vi "sub vi - calibration v1.vi"() -> ()   [LabVIEW 2013]
uses:
  <vilib>/Platform/TimedLoop/XDataNode/timing_clust.ctl
  <vilib>/Platform/TimedLoop/XDataNode/nitl_modes.ctl
  <vilib>/Platform/TimedLoop/XDataNode/wakeup.ctl
  <vilib>/platform/TimedLoop/XDataNode/XDataNode.xnode
  <vilib>/Platform/TimedLoop/XDataNode/XDNodeRunTimeDep.lvlib
panel:
  out "UPDATE":bool
  in  "stop":bool
  in  "Tab Control":T1(tab)
  out "LAB01-1 (GRAPH)":dynamicdata(graph)
  out "LAB01-2 (GRAPH)":dynamicdata(graph)
  in  "LAB01 (CAL)":T2 {"2 (TN) cal" min=0.0 step=0.01 format="%.2f"; "2 (TL) cal" min=0.0 step=0.01 format="%.2f"; "2 (PF) cal" min=0.0 step=0.01 format="%.2f"; "2 (V) cal" min=0.0 step=0.01 format="%.2f"; "2 (A) cal" min=0.0 step=0.01 format="%.2f"; "1 (TN) cal" min=0.0 step=0.01 format="%.2f"; "1 (TL) cal" min=0.0 step=0.01 format="%.2f"; "1 (PF) cal" min=0.0 step=0.01 format="%.2f"; "1 (V) cal" min=0.0 step=0.01 format="%.2f"; "1  (A) cal" min=0.0 step=0.01 format="%.2f"}
  out "LAB01 (SIGNALS)":T3 {"2 (PF)" format="%.2f"; "2 (A)" format="%.1f"; "1 (PF)" format="%.2f"; "1 (A)" format="%.1f"}
  out "LAB02 (SIGNALS)":T3 {"2 (PF)" format="%.2f"; "2 (A)" format="%.1f"; "1 (PF)" format="%.2f"; "1 (A)" format="%.1f"}
  in  "LAB02 (CAL)":T4 {"2 (TN) cal" min=0.0 step=0.01 format="%.2f"; "2 (TL) cal" min=0.0 step=0.01 format="%.2f"; "2 (PF) cal" min=0.0 step=0.01 format="%.2f"; "2 (V) cal" min=0.0 step=0.01 format="%.2f"; "2 (A) cal" min=0.0 step=0.01 format="%.2f"; "1 (TN) cal" min=0.0 step=0.01 format="%.2f"; "1 (TL) cal" min=0.0 step=0.01 format="%.2f"; "1 (PF) cal" min=0.0 step=0.01 format="%.2f"; "1 (V) cal" min=0.0 step=0.01 format="%.2f"; "1 (A) cal" min=0.0 step=0.01 format="%.2f"}
  out "LAB02-2 (GRAPH)":dynamicdata(graph)
  out "LAB02-1 (GRAPH)":dynamicdata(graph)
  out "LAB03 (SIGNALS)":T3 {"2 (PF)" format="%.2f"; "2 (A)" format="%.1f"; "1 (PF)" format="%.2f"; "1 (A)" format="%.1f"}
  in  "LAB03 (CAL)":T2 {"2 (TN) cal" min=0.0 step=0.01 format="%.2f"; "2 (TL) cal" min=0.0 step=0.01 format="%.2f"; "2 (PF) cal" min=0.0 step=0.01 format="%.2f"; "2 (V) cal" min=0.0 step=0.01 format="%.2f"; "2 (A) cal" min=0.0 step=0.01 format="%.2f"; "1 (TN) cal" min=0.0 step=0.01 format="%.2f"; "1 (TL) cal" min=0.0 step=0.01 format="%.2f"; "1 (PF) cal" min=0.0 step=0.01 format="%.2f"; "1 (V) cal" min=0.0 step=0.01 format="%.2f"; "1  (A) cal" min=0.0 step=0.01 format="%.2f"}
  out "LAB03-2 (GRAPH)":dynamicdata(graph)
  out "LAB03-1 (GRAPH)":dynamicdata(graph)
  out "LAB04 (SIGNALS)":T3 {"2 (PF)" format="%.2f"; "2 (A)" format="%.1f"; "1 (PF)" format="%.2f"; "1 (A)" format="%.1f"}
  in  "LAB04 (CAL)":T2 {"2 (TN) cal" min=0.0 step=0.01 format="%.2f"; "2 (TL) cal" min=0.0 step=0.01 format="%.2f"; "2 (PF) cal" min=0.0 step=0.01 format="%.2f"; "2 (V) cal" min=0.0 step=0.01 format="%.2f"; "2 (A) cal" min=0.0 step=0.01 format="%.2f"; "1 (TN) cal" min=0.0 step=0.01 format="%.2f"; "1 (TL) cal" min=0.0 step=0.01 format="%.2f"; "1 (PF) cal" min=0.0 step=0.01 format="%.2f"; "1 (V) cal" min=0.0 step=0.01 format="%.2f"; "1  (A) cal" min=0.0 step=0.01 format="%.2f"}
  out "LAB04-2 (GRAPH)":dynamicdata(graph)
  out "LAB04-1 (GRAPH)":dynamicdata(graph)
  out "LAB05 (SIGNALS)":T3 {"2 (PF)" format="%.2f"; "2 (A)" format="%.1f"; "1 (PF)" format="%.2f"; "1 (A)" format="%.1f"}
  in  "LAB05 (CAL)":T2 {"2 (TN) cal" min=0.0 step=0.01 format="%.2f"; "2 (TL) cal" min=0.0 step=0.01 format="%.2f"; "2 (PF) cal" min=0.0 step=0.01 format="%.2f"; "2 (V) cal" min=0.0 step=0.01 format="%.2f"; "2 (A) cal" min=0.0 step=0.01 format="%.2f"; "1 (TN) cal" min=0.0 step=0.01 format="%.2f"; "1 (TL) cal" min=0.0 step=0.01 format="%.2f"; "1 (PF) cal" min=0.0 step=0.01 format="%.2f"; "1 (V) cal" min=0.0 step=0.01 format="%.2f"; "1  (A) cal" min=0.0 step=0.01 format="%.2f"}
  out "LAB05-2 (GRAPH)":dynamicdata(graph)
  out "LAB05-1 (GRAPH)":dynamicdata(graph)
  out "Temperature data error":bool
  out "file error out":errorcluster
  out "Analog Loop Time":dbl
  out "analog read ERROR":errorcluster[](array[cluster])
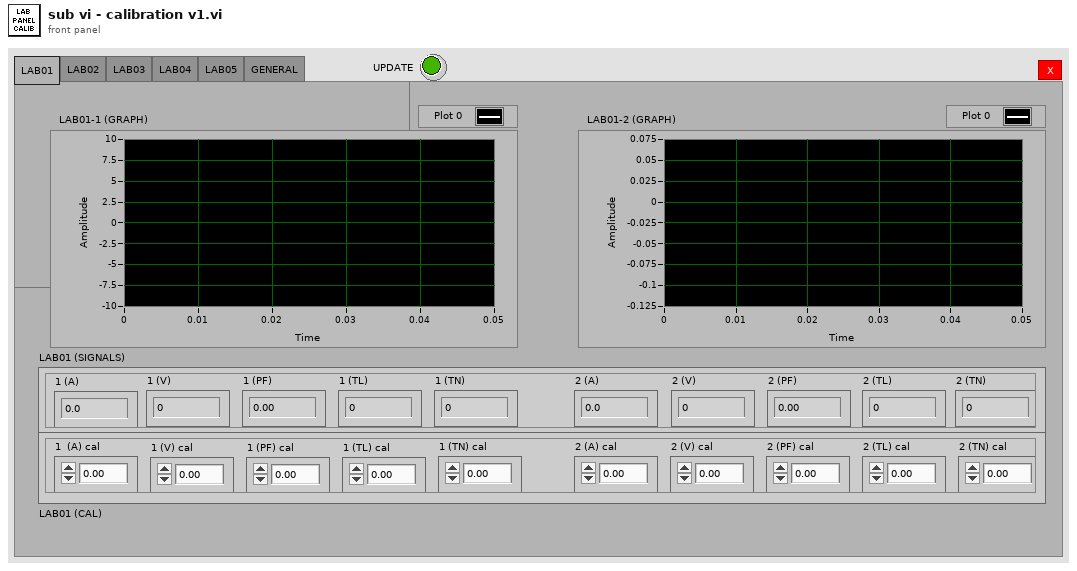
[diagram p1: front panel]
types:
  T1 = enum32{"LAB01", "LAB02", "LAB03", "LAB04", "LAB05", "GENERAL"}
  T2 = cluster{"1  (A) cal":dbl, "1 (V) cal":dbl, "1 (PF) cal":dbl, "1 (TL) cal":dbl, "1 (TN) cal":dbl, "2 (A) cal":dbl, "2 (V) cal":dbl, "2 (PF) cal":dbl, "2 (TL) cal":dbl, "2 (TN) cal":dbl}
  T3 = cluster{"1 (TL)":dbl, "1 (TN)":dbl, "2 (TL)":dbl, "2 (TN)":dbl, "1 (A)":dbl, "1 (V)":dbl, "1 (PF)":dbl, "2 (A)":dbl, "2 (V)":dbl, "2 (PF)":dbl}
  T4 = cluster{"1 (A) cal":dbl, "1 (V) cal":dbl, "1 (PF) cal":dbl, "1 (TL) cal":dbl, "1 (TN) cal":dbl, "2 (A) cal":dbl, "2 (V) cal":dbl, "2 (PF) cal":dbl, "2 (TL) cal":dbl, "2 (TN) cal":dbl}
  T5 = enum16{"open", "replace", "create", "open or create", "replace or create", "replace or create with confirmation"}
  T6 = typedef "XDNodeRunTimeDep.lvlib/timing_clust.ctl" = cluster{"Expected End [f-1]":u64, "Actual End [f-1]":u64, "Finished Late? [f-1]":bool, "Expected End [i-1]":u64, "Actual End [i-1]":u64, "Finished Late? [i-1]":bool, "Expected Start [i]":u64, "Actual Start [i]":u64, "Expected Start [f]":u64, "Actual Start [f]":u64, "Source Name":string, "Structure Name":string, "Period":i64, "Deadline":i64, "Offset":i64, "Start":i64, "Priority":i32, "Timeout":i32, "Mode":T7, "Wakeup Reason":T8, "Error":errorcluster, "Source Type":string, "Secondary Source Type":string, "Global End Time":u64, "Global Start Time":u64, "Frame Duration":u64, "Iteration Duration":u64, "Assigned CPU":i32, "I/O Scan Engine Mode":u32}
  T7 = typedef "XDNodeRunTimeDep.lvlib/nitl_modes.ctl" = enum32{"No Change", "Process missed periods, maintain original phase", "Discard missed periods, maintain original phase", "Process missed periods, ignore original phase", "Discard missed periods, ignore original phase"}
  T8 = typedef "XDNodeRunTimeDep.lvlib/wakeup.ctl" = enum32{"Normal", "Aborted", "Asynchronous wakeup", "Timing source error", "Timed loop error", "Timeout"}
  T9 = cluster{"LAB01-1 (A)":dbl, "LAB01-1 (V)":dbl, "LAB01-1 (PF)":dbl, "LAB01-2 (A)":dbl, "LAB01-2 (V)":dbl, "LAB01-2 (PF)":dbl}
  T10 = cluster{"LAB02-1 (A)":dbl, "LAB02-1 (V)":dbl, "LAB02-1 (PF)":dbl, "LAB02-2 (A)":dbl, "LAB02-2 (V)":dbl, "LAB02-2 (PF)":dbl}
  T11 = cluster{"LAB03-1 (A)":dbl, "LAB03-1 (V)":dbl, "LAB03-1 (PF)":dbl, "LAB03-2 (A)":dbl, "LAB03-2 (V)":dbl, "LAB03-2 (PF)":dbl}
  T12 = cluster{"LAB04-1 (A)":dbl, "LAB04-1 (V)":dbl, "LAB04-1 (PF)":dbl, "LAB04-2 (A)":dbl, "LAB04-2 (V)":dbl, "LAB04-2 (PF)":dbl}
  T13 = cluster{"LAB05-1 (A)":dbl, "LAB05-1 (V)":dbl, "LAB05-1 (PF)":dbl, "LAB05-2 (A)":dbl, "LAB05-2 (V)":dbl, "LAB05-2 (PF)":dbl}
  T14 = cluster{"T1":dbl, "T2":dbl, "T3":dbl, "T4":dbl, "ID":dbl, "ER":dbl}
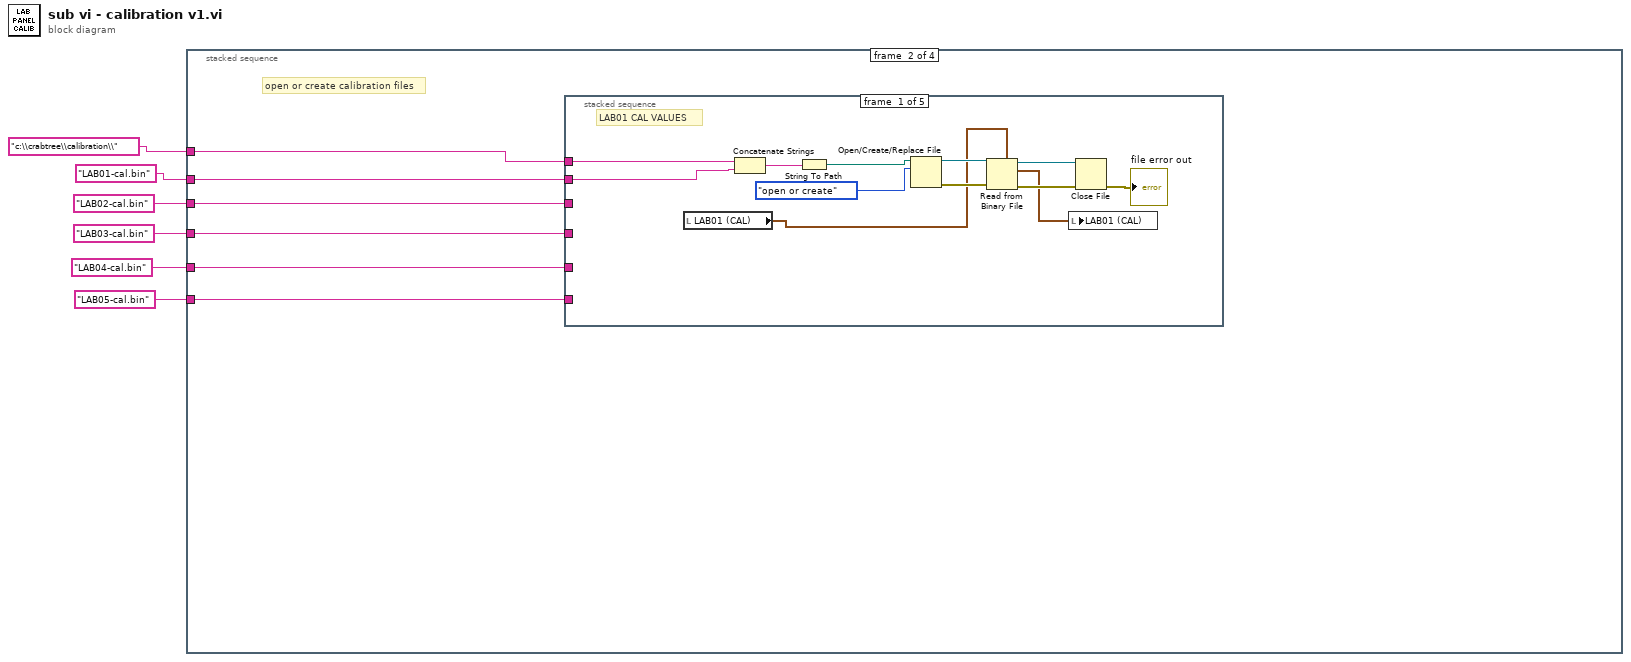
[diagram p0: block diagram]
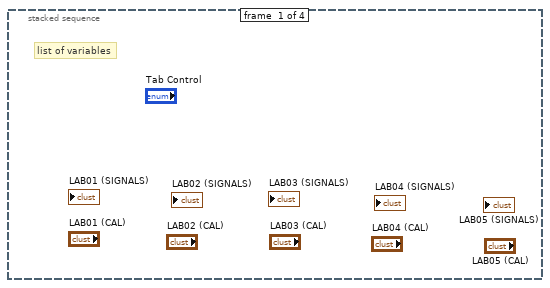
[diagram p2: hidden frame]
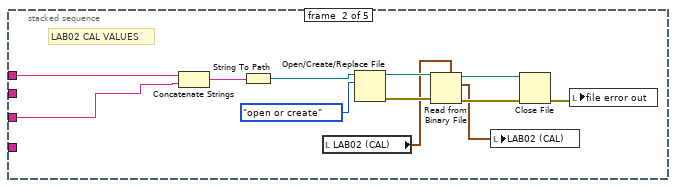
[diagram p3: hidden frame]
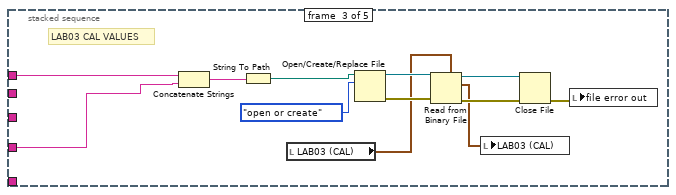
[diagram p4: hidden frame]
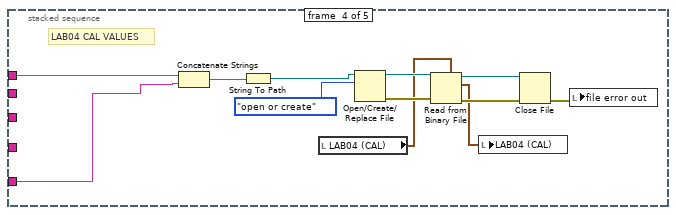
[diagram p5: hidden frame]
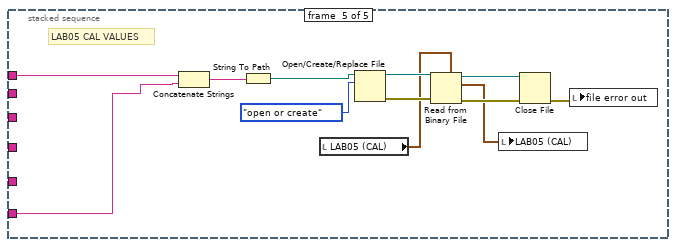
[diagram p6: hidden frame]
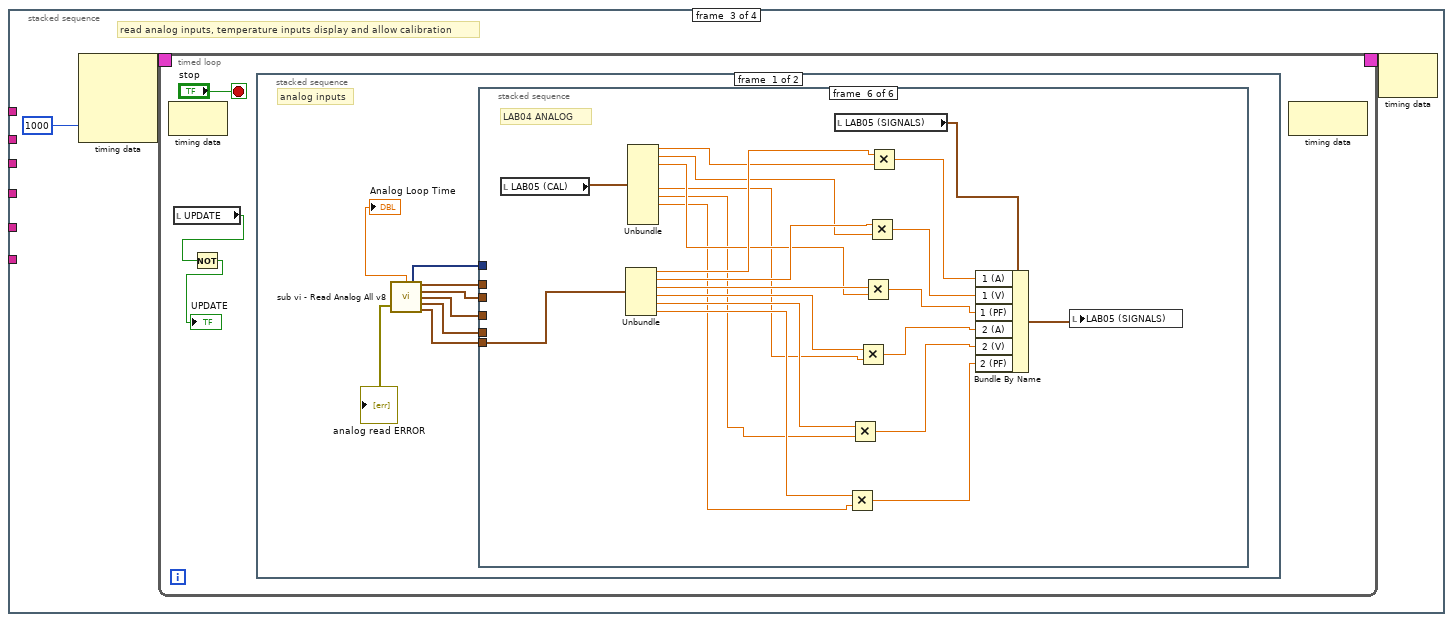
[diagram p7: hidden frame]
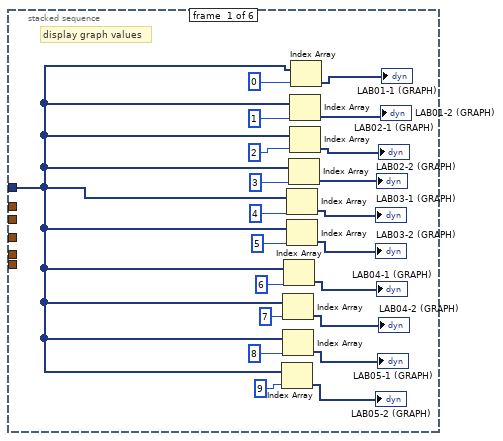
[diagram p8: hidden frame]
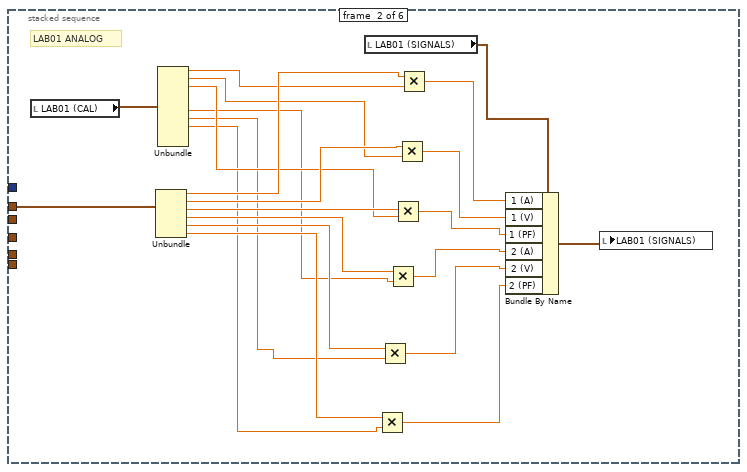
[diagram p9: hidden frame]
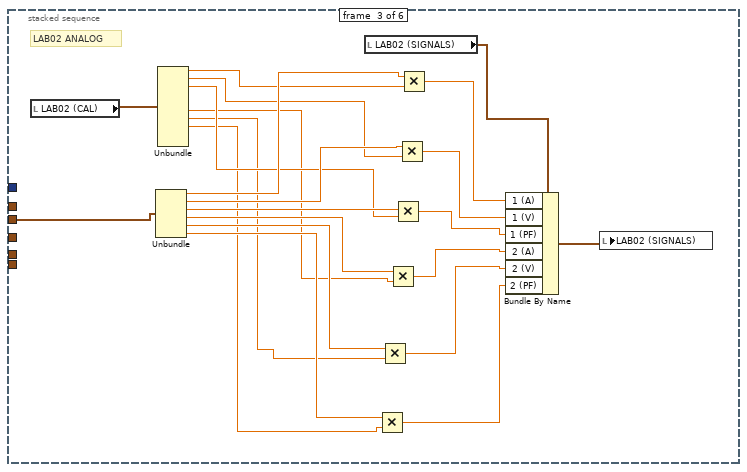
[diagram p10: hidden frame]
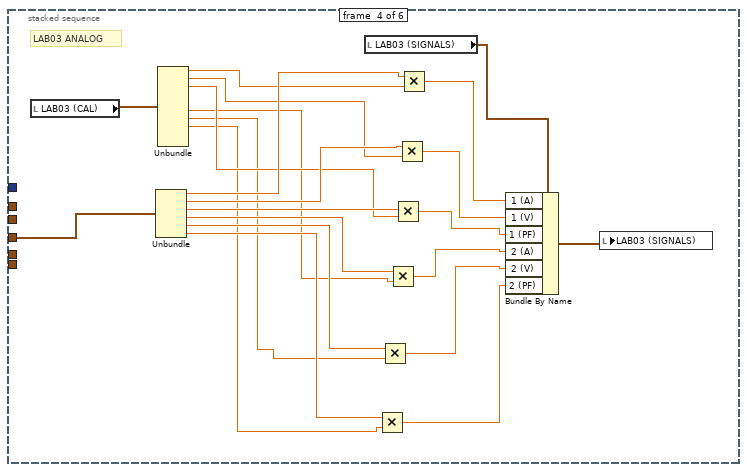
[diagram p11: hidden frame]
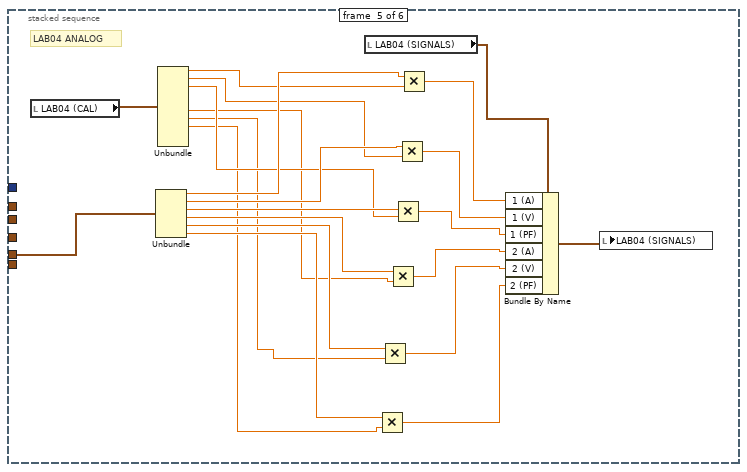
[diagram p12: hidden frame]
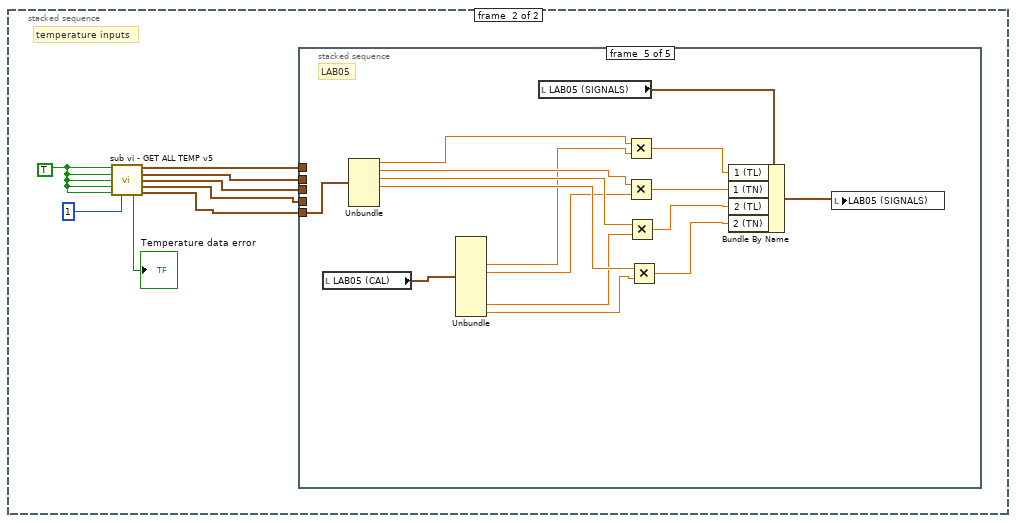
[diagram p13: hidden frame]
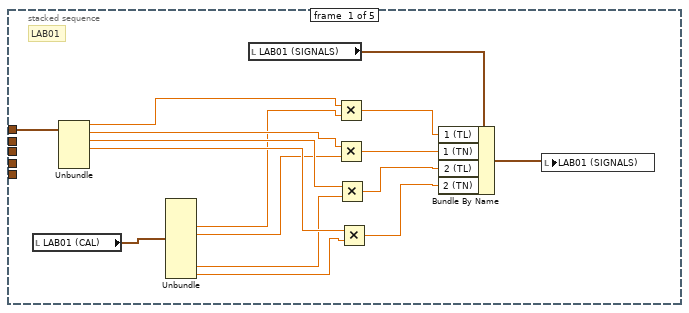
[diagram p14: hidden frame]
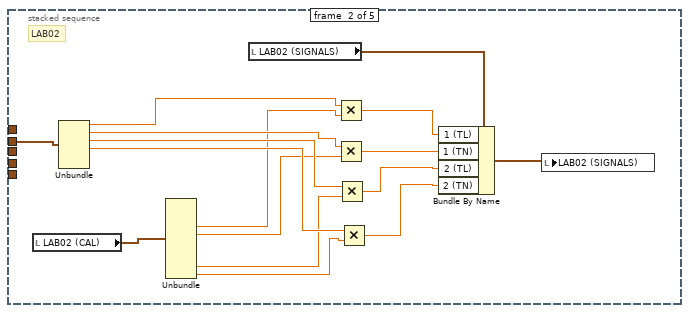
[diagram p15: hidden frame]
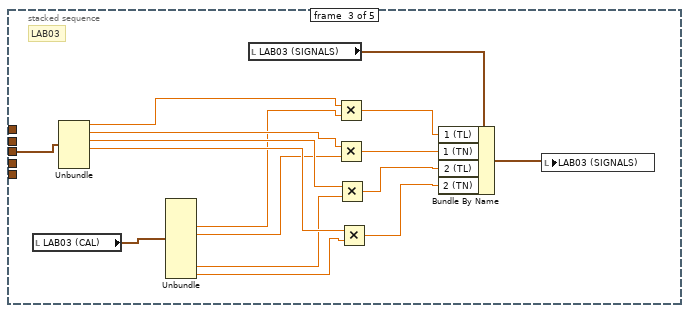
[diagram p16: hidden frame]
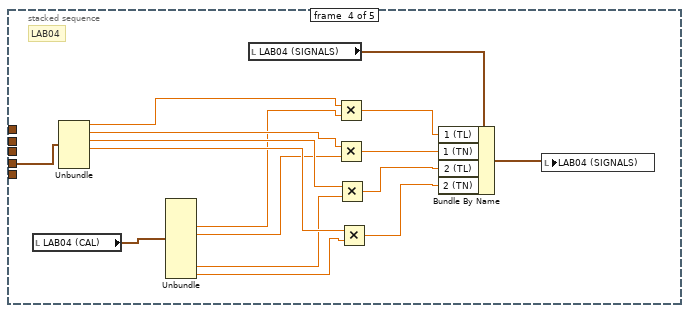
[diagram p17: hidden frame]
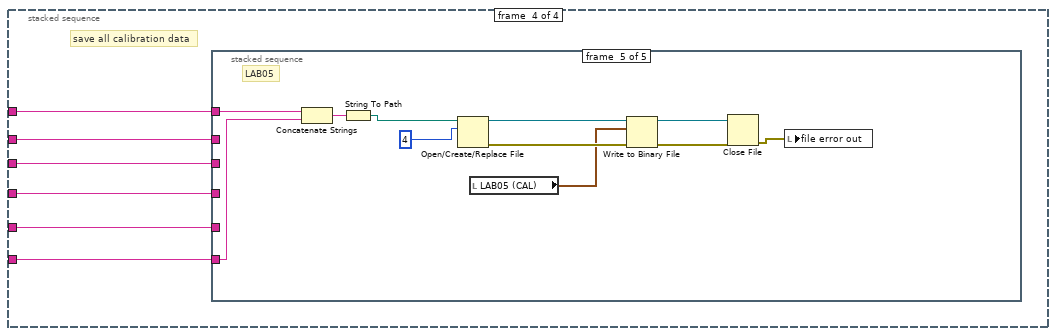
[diagram p18: hidden frame]
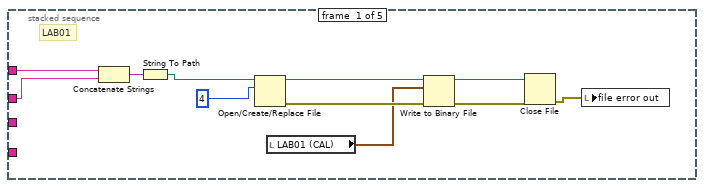
[diagram p19: hidden frame]
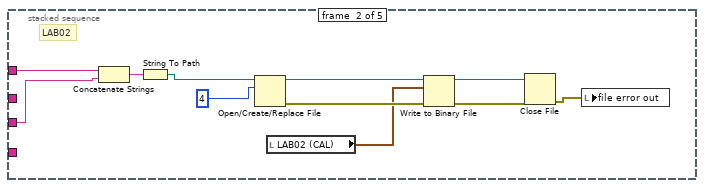
[diagram p20: hidden frame]
diagram:
  n1 = stacked-sequence {
    tunnel: "c:\\crabtree\\calibration\\" -> [_ w12 _ w317]
    tunnel: "LAB01-cal.bin" -> [_ w11 _ w316]
    tunnel: "LAB02-cal.bin" -> [_ w10 _ w315]
    tunnel: "LAB03-cal.bin" -> [_ w9 _ w314]
    tunnel: "LAB04-cal.bin" -> [_ w8 _ w313]
    tunnel: "LAB05-cal.bin" -> [_ w7 _ w312]
    frame #0 {
      # "list of variables"
    }
    frame #1 {
      # "open or create calibration files"
      n2 = stacked-sequence {
        tunnel: w12 -> [w24 w36 w48 w60 w72]
        tunnel: w11 -> [w15 _ _ _ _]
        tunnel: w10 -> [_ w27 _ _ _]
        tunnel: w9 -> [_ _ w39 _ _]
        tunnel: w8 -> [_ _ _ w52 _]
        tunnel: w7 -> [_ _ _ _ w63]
        frame #0 {
          # "LAB01 CAL VALUES"
          n3 = local read "LAB01 (CAL)"() -> (w14:T2)
          n4 = Concatenate Strings(w24, w15) -> (w23:string)
          n5 = String To Path(string=w23) -> (path=w22:path)
          n6 = Open/Create/Replace File(file path (use dialog)=w22, operation (0:open)=T5."open or create") -> (refnum out=w21:refnum<file>, error out=w20:errorcluster)  [unwired: 4 in, 1 out]
          n7 = Read from Binary File(5:w14, 8:w20, 11:w21) -> (0:w18:errorcluster, 2:w13:T2, 3:w19:refnum<file>)  [unwired: 3 in, 1 out]
          n8 = local write "LAB01 (CAL)"(w13) -> ()
          n9 = Close File(refnum=w19, error in=w18) -> (error out=→"file error out":errorcluster)  [unwired: 1 out]
        }
        frame #1 {
          # "LAB02 CAL VALUES"
          n10 = Concatenate Strings(w36, w27) -> (w35:string)
          n11 = String To Path(string=w35) -> (path=w34:path)
          n12 = local read "LAB02 (CAL)"() -> (w26:T4)
          n13 = Open/Create/Replace File(file path (use dialog)=w34, operation (0:open)=T5."open or create") -> (refnum out=w33:refnum<file>, error out=w32:errorcluster)  [unwired: 4 in, 1 out]
          n14 = Read from Binary File(5:w26, 8:w32, 11:w33) -> (0:w30:errorcluster, 2:w25:T4, 3:w31:refnum<file>)  [unwired: 3 in, 1 out]
          n15 = local write "LAB02 (CAL)"(w25) -> ()
          n16 = Close File(refnum=w31, error in=w30) -> (error out=w28:errorcluster)  [unwired: 1 out]
          n17 = local write "file error out"(w28) -> ()
        }
        frame #2 {
          # "LAB03 CAL VALUES"
          n18 = Concatenate Strings(w48, w39) -> (w47:string)
          n19 = String To Path(string=w47) -> (path=w46:path)
          n20 = local read "LAB03 (CAL)"() -> (w38:T2)
          n21 = Open/Create/Replace File(file path (use dialog)=w46, operation (0:open)=T5."open or create") -> (refnum out=w45:refnum<file>, error out=w44:errorcluster)  [unwired: 4 in, 1 out]
          n22 = Read from Binary File(5:w38, 8:w44, 11:w45) -> (0:w42:errorcluster, 2:w37:T2, 3:w43:refnum<file>)  [unwired: 3 in, 1 out]
          n23 = local write "LAB03 (CAL)"(w37) -> ()
          n24 = Close File(refnum=w43, error in=w42) -> (error out=w40:errorcluster)  [unwired: 1 out]
          n25 = local write "file error out"(w40) -> ()
        }
        frame #3 {
          # "LAB04 CAL VALUES"
          n26 = Concatenate Strings(w60, w52) -> (w59:string)
          n27 = String To Path(string=w59) -> (path=w58:path)
          n28 = local read "LAB04 (CAL)"() -> (w50:T2)
          n29 = Open/Create/Replace File(file path (use dialog)=w58, operation (0:open)=T5."open or create") -> (refnum out=w57:refnum<file>, error out=w56:errorcluster)  [unwired: 4 in, 1 out]
          n30 = Read from Binary File(5:w50, 8:w56, 11:w57) -> (0:w54:errorcluster, 2:w49:T2, 3:w55:refnum<file>)  [unwired: 3 in, 1 out]
          n31 = local write "LAB04 (CAL)"(w49) -> ()
          n32 = Close File(refnum=w55, error in=w54) -> (error out=w53:errorcluster)  [unwired: 1 out]
          n33 = local write "file error out"(w53) -> ()
        }
        frame #4 {
          # "LAB05 CAL VALUES"
          n34 = Concatenate Strings(w72, w63) -> (w71:string)
          n35 = String To Path(string=w71) -> (path=w70:path)
          n36 = local read "LAB05 (CAL)"() -> (w62:T2)
          n37 = Open/Create/Replace File(file path (use dialog)=w70, operation (0:open)=T5."open or create") -> (refnum out=w69:refnum<file>, error out=w68:errorcluster)  [unwired: 4 in, 1 out]
          n38 = Read from Binary File(5:w62, 8:w68, 11:w69) -> (0:w66:errorcluster, 2:w61:T2, 3:w67:refnum<file>)  [unwired: 3 in, 1 out]
          n39 = local write "LAB05 (CAL)"(w61) -> ()
          n40 = Close File(refnum=w67, error in=w66) -> (error out=w64:errorcluster)  [unwired: 1 out]
          n41 = local write "file error out"(w64) -> ()
        }
      }
    }
    frame #2 {
      # "read analog inputs, temperature inputs display and allow calibration"
      n42 = node-c288(1000) -> (w75:T6)  [unwired: 3 in]
      n43 = timed-loop {
        timing: w75 -> [_]
        timing-out: [_] -> w74
        stop <- "stop" stop-if-true
        n44 = node-c288() -> ()  [unwired: 1 in, 1 out]
        n45 = local read "UPDATE"() -> (w76:bool)
        n46 = Not(x=w76) -> (.not. x?=→"UPDATE":bool)
        n47 = stacked-sequence {
          frame #0 {
            # "analog inputs"
            n48 = call "sub vi - Read Analog All v8.vi"() -> ("Analog loop time"=→"Analog Loop Time":dbl, "array GRAPH"=w85:dynamicdata[], "LAB01"=w84:T9, "LAB02"=w82:T10, "LAB03"=w83:T11, "LAB04"=w81:T12, "array ERROR"=→"analog read ERROR":errorcluster[], "LAB05"=w80:T13)  [unwired: 8 in]
            n49 = stacked-sequence {
              tunnel: w85 -> [w106 _ _ _ _ _]
              tunnel: w84 -> [_ w128 _ _ _ _]
              tunnel: w83 -> [_ _ _ w152 _ _]
              tunnel: w82 -> [_ _ w130 _ _ _]
              tunnel: w81 -> [_ _ _ _ w174 _]
              tunnel: w80 -> [_ _ _ _ _ w196]
              frame #0 {
                # "display graph values"
                n50 = Index Array(array=w106, index=9) -> (element=→"LAB05-2 (GRAPH)":dynamicdata)
                n51 = Index Array(array=w106, index=7) -> (element=→"LAB04-2 (GRAPH)":dynamicdata)
                n52 = Index Array(array=w106, index=8) -> (element=→"LAB05-1 (GRAPH)":dynamicdata)
                n53 = Index Array(array=w106, index=6) -> (element=→"LAB04-1 (GRAPH)":dynamicdata)
                n54 = Index Array(array=w106, index=4) -> (element=→"LAB03-1 (GRAPH)":dynamicdata)
                n55 = Index Array(array=w106, index=5) -> (element=→"LAB03-2 (GRAPH)":dynamicdata)
                n56 = Index Array(array=w106, index=3) -> (element=→"LAB02-2 (GRAPH)":dynamicdata)
                n57 = Index Array(array=w106, index=1) -> (element=→"LAB01-2 (GRAPH)":dynamicdata)
                n58 = Index Array(array=w106, index=2) -> (element=→"LAB02-1 (GRAPH)":dynamicdata)
                n59 = Index Array(array=w106, index=0) -> (element=→"LAB01-1 (GRAPH)":dynamicdata)
              }
              frame #1 {
                # "LAB01 ANALOG"
                n60 = local read "LAB01 (CAL)"() -> (w129:T2)
                n61 = Unbundle(w128) -> ("LAB01-1 (A)"=w127:dbl, "LAB01-1 (V)"=w126:dbl, "LAB01-1 (PF)"=w125:dbl, "LAB01-2 (A)"=w124:dbl, "LAB01-2 (V)"=w123:dbl, "LAB01-2 (PF)"=w122:dbl)
                n62 = Unbundle(w129) -> ("1  (A) cal"=w121:dbl, "1 (V) cal"=w120:dbl, "1 (PF) cal"=w119:dbl, "2 (A) cal"=w118:dbl, "2 (V) cal"=w117:dbl, "2 (PF) cal"=w116:dbl)  [unwired: 4 out]
                n63 = local read "LAB01 (SIGNALS)"() -> (w115:T3)
                n64 = Multiply(x=w122, y=w116) -> (x*y=w109:dbl)
                n65 = Multiply(x=w123, y=w117) -> (x*y=w110:dbl)
                n66 = Multiply(x=w124, y=w118) -> (x*y=w111:dbl)
                n67 = Multiply(x=w125, y=w119) -> (x*y=w112:dbl)
                n68 = Multiply(x=w126, y=w120) -> (x*y=w113:dbl)
                n69 = Multiply(x=w127, y=w121) -> (x*y=w114:dbl)
                n70 = Bundle By Name(cluster=w115, "1 (A)"=w114, "1 (V)"=w113, "1 (PF)"=w112, "2 (A)"=w111, "2 (V)"=w110, "2 (PF)"=w109) -> (w108:T3)
                n71 = local write "LAB01 (SIGNALS)"(w108) -> ()
              }
              frame #2 {
                # "LAB02 ANALOG"
                n72 = local read "LAB02 (CAL)"() -> (w151:T4)
                n73 = Unbundle(w130) -> ("LAB02-1 (A)"=w150:dbl, "LAB02-1 (V)"=w149:dbl, "LAB02-1 (PF)"=w148:dbl, "LAB02-2 (A)"=w147:dbl, "LAB02-2 (V)"=w146:dbl, "LAB02-2 (PF)"=w145:dbl)
                n74 = Unbundle(w151) -> ("1 (A) cal"=w144:dbl, "1 (V) cal"=w143:dbl, "1 (PF) cal"=w142:dbl, "2 (A) cal"=w141:dbl, "2 (V) cal"=w140:dbl, "2 (PF) cal"=w139:dbl)  [unwired: 4 out]
                n75 = local read "LAB02 (SIGNALS)"() -> (w138:T3)
                n76 = Multiply(x=w145, y=w139) -> (x*y=w132:dbl)
                n77 = Multiply(x=w146, y=w140) -> (x*y=w133:dbl)
                n78 = Multiply(x=w147, y=w141) -> (x*y=w134:dbl)
                n79 = Multiply(x=w148, y=w142) -> (x*y=w135:dbl)
                n80 = Multiply(x=w149, y=w143) -> (x*y=w136:dbl)
                n81 = Multiply(x=w150, y=w144) -> (x*y=w137:dbl)
                n82 = Bundle By Name(cluster=w138, "1 (A)"=w137, "1 (V)"=w136, "1 (PF)"=w135, "2 (A)"=w134, "2 (V)"=w133, "2 (PF)"=w132) -> (w131:T3)
                n83 = local write "LAB02 (SIGNALS)"(w131) -> ()
              }
              frame #3 {
                # "LAB03 ANALOG"
                n84 = local read "LAB03 (CAL)"() -> (w173:T2)
                n85 = Unbundle(w152) -> ("LAB03-1 (A)"=w172:dbl, "LAB03-1 (V)"=w171:dbl, "LAB03-1 (PF)"=w170:dbl, "LAB03-2 (A)"=w169:dbl, "LAB03-2 (V)"=w168:dbl, "LAB03-2 (PF)"=w167:dbl)
                n86 = Unbundle(w173) -> ("1  (A) cal"=w166:dbl, "1 (V) cal"=w165:dbl, "1 (PF) cal"=w164:dbl, "2 (A) cal"=w163:dbl, "2 (V) cal"=w162:dbl, "2 (PF) cal"=w161:dbl)  [unwired: 4 out]
                n87 = local read "LAB03 (SIGNALS)"() -> (w160:T3)
                n88 = Multiply(x=w167, y=w161) -> (x*y=w154:dbl)
                n89 = Multiply(x=w168, y=w162) -> (x*y=w155:dbl)
                n90 = Multiply(x=w169, y=w163) -> (x*y=w156:dbl)
                n91 = Multiply(x=w170, y=w164) -> (x*y=w157:dbl)
                n92 = Multiply(x=w171, y=w165) -> (x*y=w158:dbl)
                n93 = Multiply(x=w172, y=w166) -> (x*y=w159:dbl)
                n94 = Bundle By Name(cluster=w160, "1 (A)"=w159, "1 (V)"=w158, "1 (PF)"=w157, "2 (A)"=w156, "2 (V)"=w155, "2 (PF)"=w154) -> (w153:T3)
                n95 = local write "LAB03 (SIGNALS)"(w153) -> ()
              }
              frame #4 {
                # "LAB04 ANALOG"
                n96 = local read "LAB04 (CAL)"() -> (w195:T2)
                n97 = Unbundle(w174) -> ("LAB04-1 (A)"=w194:dbl, "LAB04-1 (V)"=w193:dbl, "LAB04-1 (PF)"=w192:dbl, "LAB04-2 (A)"=w191:dbl, "LAB04-2 (V)"=w190:dbl, "LAB04-2 (PF)"=w189:dbl)
                n98 = Unbundle(w195) -> ("1  (A) cal"=w188:dbl, "1 (V) cal"=w187:dbl, "1 (PF) cal"=w186:dbl, "2 (A) cal"=w185:dbl, "2 (V) cal"=w184:dbl, "2 (PF) cal"=w183:dbl)  [unwired: 4 out]
                n99 = local read "LAB04 (SIGNALS)"() -> (w182:T3)
                n100 = Multiply(x=w189, y=w183) -> (x*y=w176:dbl)
                n101 = Multiply(x=w190, y=w184) -> (x*y=w177:dbl)
                n102 = Multiply(x=w191, y=w185) -> (x*y=w178:dbl)
                n103 = Multiply(x=w192, y=w186) -> (x*y=w179:dbl)
                n104 = Multiply(x=w193, y=w187) -> (x*y=w180:dbl)
                n105 = Multiply(x=w194, y=w188) -> (x*y=w181:dbl)
                n106 = Bundle By Name(cluster=w182, "1 (A)"=w181, "1 (V)"=w180, "1 (PF)"=w179, "2 (A)"=w178, "2 (V)"=w177, "2 (PF)"=w176) -> (w175:T3)
                n107 = local write "LAB04 (SIGNALS)"(w175) -> ()
              }
              frame #5 {
                # "LAB04 ANALOG"
                n108 = local read "LAB05 (CAL)"() -> (w217:T2)
                n109 = Unbundle(w196) -> ("LAB05-1 (A)"=w216:dbl, "LAB05-1 (V)"=w215:dbl, "LAB05-1 (PF)"=w214:dbl, "LAB05-2 (A)"=w213:dbl, "LAB05-2 (V)"=w212:dbl, "LAB05-2 (PF)"=w211:dbl)
                n110 = Unbundle(w217) -> ("1  (A) cal"=w210:dbl, "1 (V) cal"=w209:dbl, "1 (PF) cal"=w208:dbl, "2 (A) cal"=w207:dbl, "2 (V) cal"=w206:dbl, "2 (PF) cal"=w205:dbl)  [unwired: 4 out]
                n111 = local read "LAB05 (SIGNALS)"() -> (w204:T3)
                n112 = Multiply(x=w211, y=w205) -> (x*y=w198:dbl)
                n113 = Multiply(x=w212, y=w206) -> (x*y=w199:dbl)
                n114 = Multiply(x=w213, y=w207) -> (x*y=w200:dbl)
                n115 = Multiply(x=w214, y=w208) -> (x*y=w201:dbl)
                n116 = Multiply(x=w215, y=w209) -> (x*y=w202:dbl)
                n117 = Multiply(x=w216, y=w210) -> (x*y=w203:dbl)
                n118 = Bundle By Name(cluster=w204, "1 (A)"=w203, "1 (V)"=w202, "1 (PF)"=w201, "2 (A)"=w200, "2 (V)"=w199, "2 (PF)"=w198) -> (w197:T3)
                n119 = local write "LAB05 (SIGNALS)"(w197) -> ()
              }
            }
          }
          frame #1 {
            w225 = TRUE
            # "temperature inputs"
            n120 = call "sub vi - GET ALL TEMP v5.vi"("LA01-EN"=w225, "LA02-EN"=w225, "LA03-EN"=w225, "LA04-EN"=w225, "LA05-EN"=w225, "Gen Cal Value"=1) -> ("LA01 TEMP"=w223:T14, "LA02 TEMP"=w221:T14, "LA03 TEMP"=w220:T14, "LA04 TEMP"=w219:T14, "error"=→"Temperature data error":bool, "LA05 TEMP"=w218:T14)  [unwired: 4 in]
            n121 = stacked-sequence {
              tunnel: w223 -> [w240 _ _ _ _]
              tunnel: w221 -> [_ w242 _ _ _]
              tunnel: w220 -> [_ _ w258 _ _]
              tunnel: w219 -> [_ _ _ w274 _]
              tunnel: w218 -> [_ _ _ _ w290]
              frame #0 {
                # "LAB01"
                n122 = local read "LAB01 (CAL)"() -> (w241:T2)
                n123 = Unbundle(w240) -> ("T1"=w239:dbl, "T2"=w238:dbl, "T3"=w237:dbl, "T4"=w236:dbl)  [unwired: 2 out]
                n124 = Unbundle(w241) -> ("1 (TL) cal"=w235:dbl, "1 (TN) cal"=w234:dbl, "2 (TL) cal"=w233:dbl, "2 (TN) cal"=w232:dbl)  [unwired: 6 out]
                n125 = local read "LAB01 (SIGNALS)"() -> (w231:T3)
                n126 = Multiply(x=w239, y=w235) -> (x*y=w230:dbl)
                n127 = Multiply(x=w238, y=w234) -> (x*y=w229:dbl)
                n128 = Multiply(x=w237, y=w233) -> (x*y=w228:dbl)
                n129 = Multiply(x=w236, y=w232) -> (x*y=w227:dbl)
                n130 = Bundle By Name(cluster=w231, "1 (TL)"=w230, "1 (TN)"=w229, "2 (TL)"=w228, "2 (TN)"=w227) -> (w226:T3)
                n131 = local write "LAB01 (SIGNALS)"(w226) -> ()
              }
              frame #1 {
                # "LAB02"
                n132 = local read "LAB02 (CAL)"() -> (w257:T4)
                n133 = Unbundle(w242) -> ("T1"=w256:dbl, "T2"=w255:dbl, "T3"=w254:dbl, "T4"=w253:dbl)  [unwired: 2 out]
                n134 = Unbundle(w257) -> ("1 (TL) cal"=w252:dbl, "1 (TN) cal"=w251:dbl, "2 (TL) cal"=w250:dbl, "2 (TN) cal"=w249:dbl)  [unwired: 6 out]
                n135 = local read "LAB02 (SIGNALS)"() -> (w248:T3)
                n136 = Multiply(x=w256, y=w252) -> (x*y=w247:dbl)
                n137 = Multiply(x=w255, y=w251) -> (x*y=w246:dbl)
                n138 = Multiply(x=w254, y=w250) -> (x*y=w245:dbl)
                n139 = Multiply(x=w253, y=w249) -> (x*y=w244:dbl)
                n140 = Bundle By Name(cluster=w248, "1 (TL)"=w247, "1 (TN)"=w246, "2 (TL)"=w245, "2 (TN)"=w244) -> (w243:T3)
                n141 = local write "LAB02 (SIGNALS)"(w243) -> ()
              }
              frame #2 {
                # "LAB03"
                n142 = local read "LAB03 (CAL)"() -> (w273:T2)
                n143 = Unbundle(w258) -> ("T1"=w272:dbl, "T2"=w271:dbl, "T3"=w270:dbl, "T4"=w269:dbl)  [unwired: 2 out]
                n144 = Unbundle(w273) -> ("1 (TL) cal"=w268:dbl, "1 (TN) cal"=w267:dbl, "2 (TL) cal"=w266:dbl, "2 (TN) cal"=w265:dbl)  [unwired: 6 out]
                n145 = local read "LAB03 (SIGNALS)"() -> (w264:T3)
                n146 = Multiply(x=w272, y=w268) -> (x*y=w263:dbl)
                n147 = Multiply(x=w271, y=w267) -> (x*y=w262:dbl)
                n148 = Multiply(x=w270, y=w266) -> (x*y=w261:dbl)
                n149 = Multiply(x=w269, y=w265) -> (x*y=w260:dbl)
                n150 = Bundle By Name(cluster=w264, "1 (TL)"=w263, "1 (TN)"=w262, "2 (TL)"=w261, "2 (TN)"=w260) -> (w259:T3)
                n151 = local write "LAB03 (SIGNALS)"(w259) -> ()
              }
              frame #3 {
                # "LAB04"
                n152 = local read "LAB04 (CAL)"() -> (w289:T2)
                n153 = Unbundle(w274) -> ("T1"=w288:dbl, "T2"=w287:dbl, "T3"=w286:dbl, "T4"=w285:dbl)  [unwired: 2 out]
                n154 = Unbundle(w289) -> ("1 (TL) cal"=w284:dbl, "1 (TN) cal"=w283:dbl, "2 (TL) cal"=w282:dbl, "2 (TN) cal"=w281:dbl)  [unwired: 6 out]
                n155 = local read "LAB04 (SIGNALS)"() -> (w280:T3)
                n156 = Multiply(x=w288, y=w284) -> (x*y=w279:dbl)
                n157 = Multiply(x=w287, y=w283) -> (x*y=w278:dbl)
                n158 = Multiply(x=w286, y=w282) -> (x*y=w277:dbl)
                n159 = Multiply(x=w285, y=w281) -> (x*y=w276:dbl)
                n160 = Bundle By Name(cluster=w280, "1 (TL)"=w279, "1 (TN)"=w278, "2 (TL)"=w277, "2 (TN)"=w276) -> (w275:T3)
                n161 = local write "LAB04 (SIGNALS)"(w275) -> ()
              }
              frame #4 {
                # "LAB05"
                n162 = local read "LAB05 (CAL)"() -> (w305:T2)
                n163 = Unbundle(w290) -> ("T1"=w304:dbl, "T2"=w303:dbl, "T3"=w302:dbl, "T4"=w301:dbl)  [unwired: 2 out]
                n164 = Unbundle(w305) -> ("1 (TL) cal"=w300:dbl, "1 (TN) cal"=w299:dbl, "2 (TL) cal"=w298:dbl, "2 (TN) cal"=w297:dbl)  [unwired: 6 out]
                n165 = local read "LAB05 (SIGNALS)"() -> (w296:T3)
                n166 = Multiply(x=w304, y=w300) -> (x*y=w295:dbl)
                n167 = Multiply(x=w303, y=w299) -> (x*y=w294:dbl)
                n168 = Multiply(x=w302, y=w298) -> (x*y=w293:dbl)
                n169 = Multiply(x=w301, y=w297) -> (x*y=w292:dbl)
                n170 = Bundle By Name(cluster=w296, "1 (TL)"=w295, "1 (TN)"=w294, "2 (TL)"=w293, "2 (TN)"=w292) -> (w291:T3)
                n171 = local write "LAB05 (SIGNALS)"(w291) -> ()
              }
            }
          }
        }
        n172 = node-c288() -> ()  [unwired: 1 in, 1 out]
      }
      n173 = node-c288(w74) -> ()  [unwired: 1 out]
    }
    frame #3 {
      # "save all calibration data"
      n174 = stacked-sequence {
        tunnel: w317 -> [w327 w338 w349 w360 w371]
        tunnel: w316 -> [w326 _ _ _ _]
        tunnel: w315 -> [_ w329 _ _ _]
        tunnel: w314 -> [_ _ w340 _ _]
        tunnel: w313 -> [_ _ _ w351 _]
        tunnel: w312 -> [_ _ _ _ w362]
        frame #0 {
          # "LAB01"
          n175 = Concatenate Strings(w327, w326) -> (w328:string)
          n176 = String To Path(string=w328) -> (path=w325:path)
          n177 = Open/Create/Replace File(file path (use dialog)=w325, operation (0:open)=4) -> (refnum out=w324:refnum<file>, error out=w323:errorcluster)  [unwired: 4 in, 1 out]
          n178 = local read "LAB01 (CAL)"() -> (w318:T2)
          n179 = Write to Binary File(file (use dialog)=w324, data=w318, error in=w323) -> (refnum out=w322:refnum<file>, error out=w321:errorcluster)  [unwired: 3 in, 1 out]
          n180 = Close File(refnum=w322, error in=w321) -> (error out=w320:errorcluster)  [unwired: 1 out]
          n181 = local write "file error out"(w320) -> ()
        }
        frame #1 {
          # "LAB02"
          n182 = Concatenate Strings(w338, w329) -> (w339:string)
          n183 = String To Path(string=w339) -> (path=w337:path)
          n184 = Open/Create/Replace File(file path (use dialog)=w337, operation (0:open)=4) -> (refnum out=w336:refnum<file>, error out=w335:errorcluster)  [unwired: 4 in, 1 out]
          n185 = local read "LAB02 (CAL)"() -> (w330:T4)
          n186 = Write to Binary File(file (use dialog)=w336, data=w330, error in=w335) -> (refnum out=w334:refnum<file>, error out=w333:errorcluster)  [unwired: 3 in, 1 out]
          n187 = Close File(refnum=w334, error in=w333) -> (error out=w332:errorcluster)  [unwired: 1 out]
          n188 = local write "file error out"(w332) -> ()
        }
        frame #2 {
          # "LAB03"
          n189 = Concatenate Strings(w349, w340) -> (w350:string)
          n190 = String To Path(string=w350) -> (path=w348:path)
          n191 = Open/Create/Replace File(file path (use dialog)=w348, operation (0:open)=4) -> (refnum out=w347:refnum<file>, error out=w346:errorcluster)  [unwired: 4 in, 1 out]
          n192 = local read "LAB03 (CAL)"() -> (w341:T2)
          n193 = Write to Binary File(file (use dialog)=w347, data=w341, error in=w346) -> (refnum out=w345:refnum<file>, error out=w344:errorcluster)  [unwired: 3 in, 1 out]
          n194 = Close File(refnum=w345, error in=w344) -> (error out=w343:errorcluster)  [unwired: 1 out]
          n195 = local write "file error out"(w343) -> ()
        }
        frame #3 {
          # "LAB04"
          n196 = Concatenate Strings(w360, w351) -> (w361:string)
          n197 = String To Path(string=w361) -> (path=w359:path)
          n198 = Open/Create/Replace File(file path (use dialog)=w359, operation (0:open)=4) -> (refnum out=w358:refnum<file>, error out=w357:errorcluster)  [unwired: 4 in, 1 out]
          n199 = local read "LAB04 (CAL)"() -> (w352:T2)
          n200 = Write to Binary File(file (use dialog)=w358, data=w352, error in=w357) -> (refnum out=w356:refnum<file>, error out=w355:errorcluster)  [unwired: 3 in, 1 out]
          n201 = Close File(refnum=w356, error in=w355) -> (error out=w354:errorcluster)  [unwired: 1 out]
          n202 = local write "file error out"(w354) -> ()
        }
        frame #4 {
          # "LAB05"
          n203 = Concatenate Strings(w371, w362) -> (w372:string)
          n204 = String To Path(string=w372) -> (path=w370:path)
          n205 = Open/Create/Replace File(file path (use dialog)=w370, operation (0:open)=4) -> (refnum out=w369:refnum<file>, error out=w368:errorcluster)  [unwired: 4 in, 1 out]
          n206 = local read "LAB05 (CAL)"() -> (w363:T2)
          n207 = Write to Binary File(file (use dialog)=w369, data=w363, error in=w368) -> (refnum out=w367:refnum<file>, error out=w366:errorcluster)  [unwired: 3 in, 1 out]
          n208 = Close File(refnum=w367, error in=w366) -> (error out=w365:errorcluster)  [unwired: 1 out]
          n209 = local write "file error out"(w365) -> ()
        }
      }
    }
  }
